vi "Fetch Measurement (Multiple).vi"(8 "error in (no error)":errorcluster, 9 "Timeout (10000 ms)":i32=10000, 10 "Number of Measurements (1)":i32=1, 11 "VISA resource name":refnum<visa-resource-name>) -> (0 "error out":errorcluster, 2 "Measurements":dbl[](array[numeric]), 3 "VISA resource name out":refnum<visa-resource-name>)   [LabVIEW 2019, in "Pendulum CNT90.lvlib"]
doc: "The fetch array query retrieves array of measuring results from the measurement result buffer of the counter without making new measurements.\n\n<B>Note</B> This VI does not check the instrument status. Typically, you call this VI only in a sequence of calls to other low-level instrument driver VIs. The sequence performs one operation. You use the low-level VIs to optimize one or more aspects of interaction with the instrument."
uses:
  Pendulum CNT90.lvlib
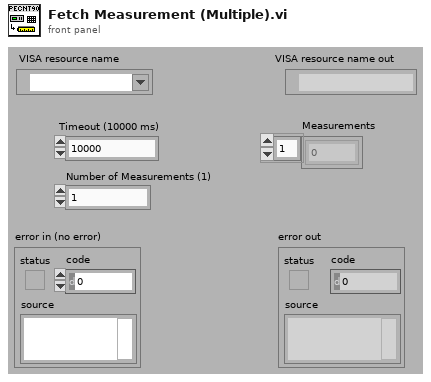
[diagram p1: front panel]
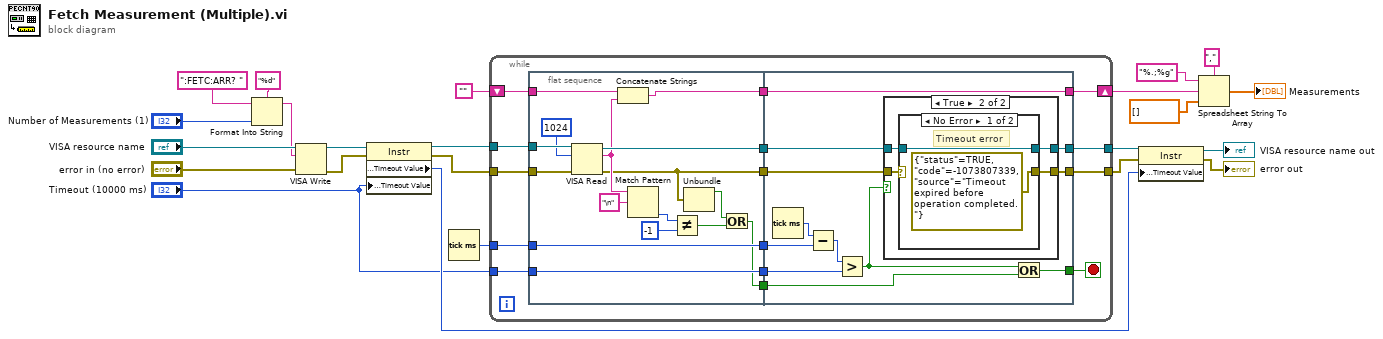
[diagram p0: block diagram]
diagram:
  n1 = Format Into String(format string="%d", initial string=":FETC:ARR? " ("write buffer"), "Number of Measurements (1)") -> (resulting string=w3:string)  [unwired: 1 in, 1 out]
  n2 = VISA Write(VISA resource name="VISA resource name", write buffer=w3, error in (no error)="error in (no error)") -> (VISA resource name out=w17:refnum<visa-resource-name>, error out=w23:errorcluster)  [unwired: 1 out]
  n3 = property class="Instr"(reference=w17, error in=w23, "General Settings:Timeout Value"="Timeout (10000 ms)") -> (reference out=w16:refnum<visa-resource-name>, error out=w22:errorcluster, "General Settings:Timeout Value"=w18:u32)
  n4 = Tick Count (ms)() -> (millisecond timer value=w6:u32)
  n5 = while {
    tunnel: w22 -> [w38]
    tunnel: [w37] -> w21
    tunnel: w16 -> [w36]
    tunnel: [w33] -> w13
    shift-right: [w34] -> w7
    shift-left: "" -> [w35]
    tunnel: w6 -> [w28]
    tunnel: "Timeout (10000 ms)" -> [w27]
    stop <- w24 stop-if-true
    n6 = flat-sequence {
      tunnel: w38 -> [w54]
      tunnel: w36 -> [w52]
      tunnel: w35 -> [w50]
      tunnel: [w53] -> w32
      tunnel: [w49] -> w31
      tunnel: [w44] -> w30
      tunnel: [w42] -> w29
      tunnel: w28 -> [w42]
      tunnel: w27 -> [w41]
      tunnel: [w41] -> w26
      tunnel: [w39] -> w25
      tunnel: [w61] -> w33
      tunnel: [w66] -> w34
      tunnel: [w58] -> w37
      tunnel: w32 -> [w59]
      tunnel: w31 -> [w66]
      tunnel: w30 -> [w60]
      tunnel: w29 -> [w64]
      tunnel: w26 -> [w62]
      tunnel: w25 -> [w57]
      tunnel: [w55] -> w24
      frame #0 {
        n7 = VISA Read(VISA resource name=w52, byte count=u32 1024, error in (no error)=w54) -> (VISA resource name out=w53:refnum<visa-resource-name>, read buffer=w48:string, error out=w44:errorcluster)  [unwired: 1 out]
        n8 = Concatenate Strings(w50, w48) -> (w49:string)
        n9 = Match Pattern(string=w48, regular expression="\n") -> (offset past match=w47:i32)  [unwired: 1 in, 3 out]
        n10 = Not Equal?(x=w47, y=-1) -> (x != y?=w43:bool)
        n11 = Unbundle(w44) -> ("status"=w40:bool)  [unwired: 2 out]
        n12 = Or(x=w40, y=w43) -> (x .or. y?=w39:bool)
      }
      frame #1 {
        n13 = Tick Count (ms)() -> (millisecond timer value=w65:u32)
        n14 = Subtract(x=w65, y=w64) -> (x-y=w63:u32)
        n15 = Greater?(x=w63, y=w62) -> (0:w56:bool)
        n16 = case shown="True" w56 {
          tunnel: [w68 w72] -> w61
          tunnel: w60 -> [w68 w69]
          tunnel: w59 -> [w67 w71]
          tunnel: [w67 w70] -> w58
          frame False {
          }
          frame True {
            n17 = case shown="No Error" w69 {
              selector: w69 -> [_ w75]
              tunnel: [errorcluster {"status"=TRUE, "code"=-1073807339, "source"="Timeout expired before operation completed."} ("error out") w75] -> w72
              tunnel: w71 -> [w73 w76]
              tunnel: [w73 w76] -> w70
              frame No Error {
                # "Timeout error"
              }
              frame Error {
              }
            }
          }
        }
        n18 = Or(x=w56, y=w57) -> (x .or. y?=w55:bool)
      }
    }
  }
  n19 = property class="Instr"(reference=w21, error in=w13, "General Settings:Timeout Value"=w18) -> (reference out=→"VISA resource name out":refnum<visa-resource-name>, error out=→"error out":errorcluster)
  n20 = Spreadsheet String To Array(delimiter (Tab)=",", format string="%.;%g", spreadsheet string=w7, array type (2D Dbl)=dbl[] [] ("Results")) -> (array=→"Measurements":dbl[])
